vi "Service Selected.vi"(8 "error in (no error)":errorcluster, 10 "Wash Car Cost":T1(array[cluster]) {"Cost" format="$ %.1f"}, 11 "Paquetes Disponibles in":refnum<class "Paquetes Disponibles.lvclass">) -> (0 "error out":errorcluster, 3 "Paquetes Disponibles out":refnum<class "Paquetes Disponibles.lvclass">)   [LabVIEW 2020, in "Paquetes Disponibles.lvlib" / "Paquetes Disponibles.lvclass"]
uses:
  Paquetes Disponibles.lvclass
  C:/Program Files (x86)/National Instruments/LabVIEW 2020/vi.lib/ActorFramework/Actor/Actor.lvclass
  <vilib>/ActorFramework/Actor/Actor.lvclass/Actor.ctl
  Paquetes Disponibles.lvclass/Paquetes Disponibles.ctl
  User Interface Messages/Cost manage Msg/Cost manage Msg.lvclass/Cost manage Msg.ctl
  <vilib>/ActorFramework/Message Enqueuer/Message Enqueuer.lvclass/Message Enqueuer.ctl
  <vilib>/ActorFramework/Message Enqueuer/Enqueue.vi
  User Interface Messages/Cost manage Msg/Cost manage Msg.lvclass
  C:/Program Files (x86)/National Instruments/LabVIEW 2020/vi.lib/ActorFramework/Message/Message.lvclass
  User Interface Messages/Load inventory Msg/Load inventory Msg.lvclass
  <vilib>/ActorFramework/Message Priority Queue/Priority Enqueue.vi
  <vilib>/ActorFramework/Actor/Actor.lvclass
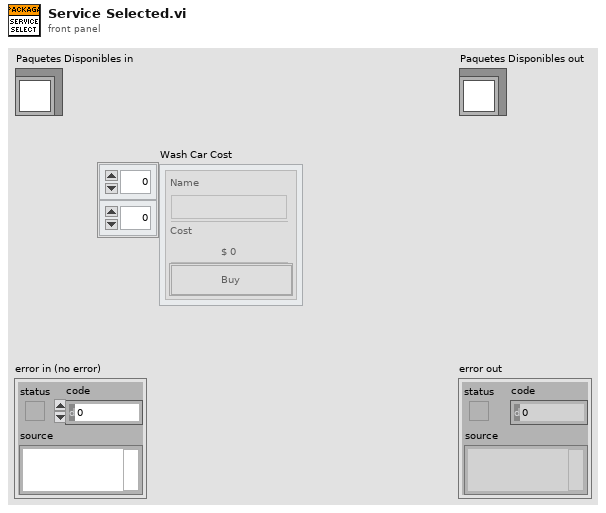
[diagram p1: front panel]
types:
  T1 = cluster{"Name":string, "Cost":u8, "Comprar":bool}[][]
  T2 = cluster{"Name":string, "Cost":u8, "Comprar":bool}[]
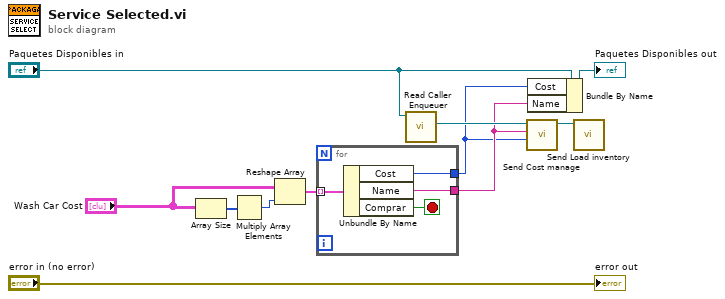
[diagram p0: block diagram]
diagram:
  n1 = Array Size(array="Wash Car Cost") -> (size(s)=w8:i32[])
  n2 = Multiply Array Elements(1:w8) -> (0:w9:i32)
  n3 = Reshape Array("Wash Car Cost", w9) -> (w10:T2)
  n4 = for {
    tunnel: w10 -> [w13] mode=indexing
    tunnel: [w15] -> w3
    tunnel: [w14] -> w2
    stop <- w12 stop-if-true
    n5 = Unbundle By Name(w13) -> ("Cost"=w14:u8, "Name"=w15:string, "Comprar"=w12:bool)
  }
  n6 = call <vilib>:"Read Caller Enqueuer.vi"("Actor"="Paquetes Disponibles in") -> ("Caller Enqueuer"=w4:refnum<class "Message Enqueuer.lvclass">)  [unwired: 10 in]
  n7 = call "Send Cost manage.vi"("Cost"=w2, "Name"=w3, "Message Enqueuer"=w4) -> ("Message Enqueuer out"=w1:refnum<class "Message Enqueuer.lvclass">)  [unwired: 7 in, 1 out]
  n8 = Bundle By Name(cluster="Paquetes Disponibles in", "Cost"=w2, "Name"=w3) -> (→"Paquetes Disponibles out":refnum<class "Paquetes Disponibles.lvclass">)
  n9 = call "Send Load inventory.vi"("Message Enqueuer"=w1) -> ()  [unwired: 9 in, 2 out]
  "error out" <- "error in (no error)"
